vi "Sec_to_date_filename.vi"(9 "ss1904":dbl) -> (1 "shortMonthName":string, 2 "shortDayName":string, 3 "HH:MM":string, 4 "YYYY":string, 6 "mm-YYYY":string, 8 "DD":string, 10 "DD-mm-YYYY":string, 12 "YYYY-mm-DD":string, 14 "YYYY-mm-DD HH:MM":string, 15 "localisedTime":string)   [LabVIEW 2020]
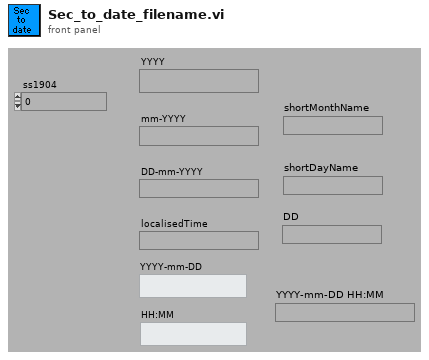
[diagram p1: front panel]
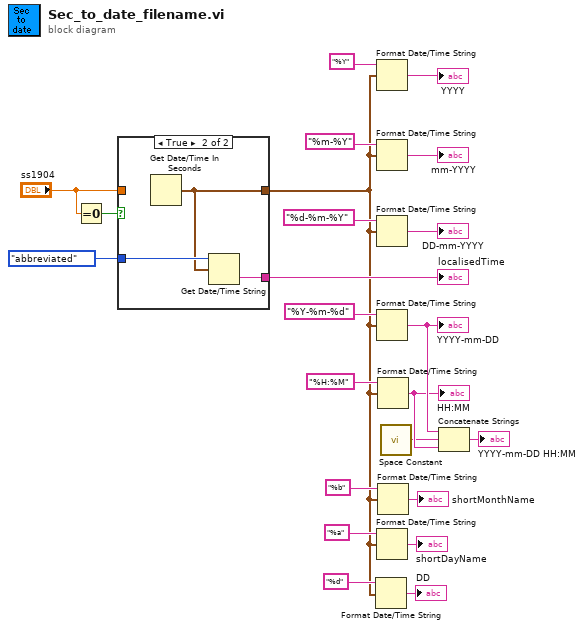
[diagram p0: block diagram]
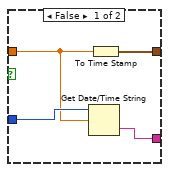
[diagram p2: hidden frame]
diagram:
  n1 = Equal To 0?(x="ss1904") -> (x = 0?=w23:bool)
  n2 = case shown="True" w23 {
    tunnel: "ss1904" -> [w24 _]
    tunnel: [w27 w30] -> w21
    tunnel: enum16{"short", "long", "abbreviated"}."abbreviated" ("date format (0)") -> [w26 w29]
    tunnel: [w25 w28] -> w1
    frame False {
      n3 = Get Date/Time String(date format (0)=w26, seconds (now)=w24) -> (time string=w27:string)  [unwired: 2 out]
      n4 = To Time Stamp(1:w24) -> (0:w25:timestamp)
    }
    frame True {
      n5 = Get Date/Time In Seconds() -> (seconds since 1Jan1904=w28:timestamp)
      n6 = Get Date/Time String(date format (0)=w29, seconds (now)=w28) -> (time string=w30:string)  [unwired: 2 out]
    }
  }
  "localisedTime" <- w21
  n7 = Format Date/Time String(time format string (%c)="%d", seconds (now)=w1) -> (date/time string=→"DD":string)  [unwired: 1 in]
  n8 = Format Date/Time String(time format string (%c)="%Y", seconds (now)=w1) -> (date/time string=→"YYYY":string)  [unwired: 1 in]
  n9 = Format Date/Time String(time format string (%c)="%m-%Y", seconds (now)=w1) -> (date/time string=→"mm-YYYY":string)  [unwired: 1 in]
  n10 = Format Date/Time String(time format string (%c)="%d-%m-%Y", seconds (now)=w1) -> (date/time string=→"DD-mm-YYYY":string)  [unwired: 1 in]
  n11 = Format Date/Time String(time format string (%c)="%Y-%m-%d", seconds (now)=w1) -> (date/time string=w11:string)  [unwired: 1 in]
  "YYYY-mm-DD" <- w11
  n12 = Format Date/Time String(time format string (%c)="%a", seconds (now)=w1) -> (date/time string=→"shortDayName":string)  [unwired: 1 in]
  n13 = Format Date/Time String(time format string (%c)="%H:%M", seconds (now)=w1) -> (date/time string=w10:string)  [unwired: 1 in]
  "HH:MM" <- w10
  n14 = Format Date/Time String(time format string (%c)="%b", seconds (now)=w1) -> (date/time string=→"shortMonthName":string)  [unwired: 1 in]
  n15 = call <vilib>:"Space Constant.vi"() -> ("String"=w9:string)
  n16 = Concatenate Strings(w11, w9, w10) -> (→"YYYY-mm-DD HH:MM":string)
